vi "xy data pinning.vi"(0 "X-Axis Array input":dbl[][](array[numeric])=array1025x10[10250 elements] format="%.2f", 1 "Data Array Input":dbl[][](array[numeric])=array1025x10[10250 elements] format="%.2f", 2 "Changed Pinning?":bool[](array[boolean]), 4 "Pinned Column #":i8=7) -> (5 "X-Axis Array output":dbl[][](array[numeric]) format="%.2f", 6 "Data Array output":dbl[][](array[numeric]) format="%.2f")   [LabVIEW 2019]
panel:
  out "where":i8
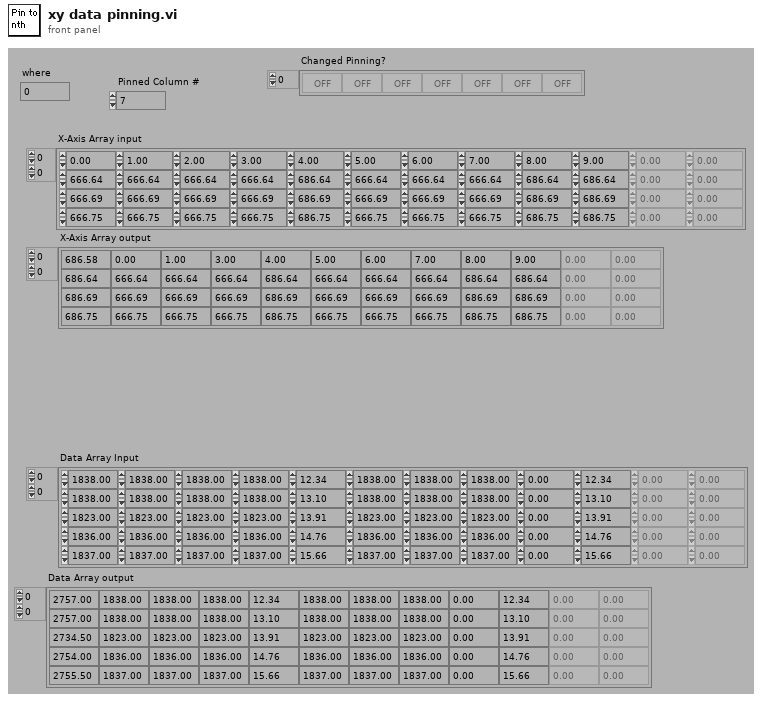
[diagram p1: front panel]
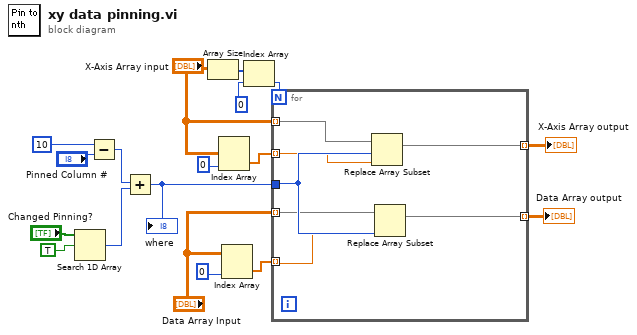
[diagram p0: block diagram]
diagram:
  n1 = Search 1D Array(1D array="Changed Pinning?", element=TRUE) -> (index of element=w9:i32)  [unwired: 1 in]
  n2 = Subtract(x=10, y="Pinned Column #") -> (x-y=w10:i32)
  n3 = Add(x=w10, y=w9) -> (x+y=w8:i32)
  "where" <- w8
  n4 = Array Size(array="X-Axis Array input") -> (size(s)=w17:i32[])
  n5 = Index Array(array="X-Axis Array input", index (col)=0) -> (element=w16:dbl[])  [unwired: 1 in]
  n6 = Index Array(array="Data Array Input", index (col)=0) -> (element=w15:dbl[])  [unwired: 1 in]
  n7 = Index Array(array=w17, index=0) -> (element=w4:i32)
  n8 = for {
    N: w4 -> [_]
    tunnel: w16 -> [w19] mode=indexing
    tunnel: w8 -> [w24]
    tunnel: "X-Axis Array input" -> [w25] mode=indexing
    tunnel: w15 -> [w23] mode=indexing
    tunnel: "Data Array Input" -> [w22] mode=indexing
    tunnel: [w21] -> w7 mode=indexing
    tunnel: [w20] -> w3 mode=indexing
    n9 = Replace Array Subset(array=w25, new element=w19, index=w24) -> (w21:dbl[])
    n10 = Replace Array Subset(array=w22, new element=w23, index=w24) -> (w20:dbl[])
  }
  "Data Array output" <- w3
  "X-Axis Array output" <- w7
